vi "GameDataToFieldState.vi"(1 "Game Data":T1={"Close  Switch"=enum."Right", "Scale"=enum."Right", "Far Switch"=enum."Right"}) -> (0 "FieldState":T3)   [LabVIEW 2017]
uses:
  TypeDef/AutoFieldState.ctl
  TypeDef/Game_Data.ctl
  TypeDef/Plate_Positions.ctl
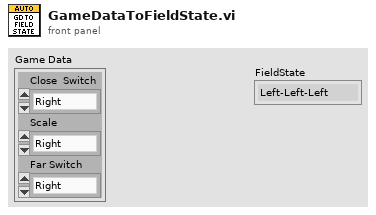
[diagram p1: front panel]
types:
  T1 = typedef "Game_Data.ctl" = cluster{"Close  Switch":T2, "Scale":T2, "Far Switch":T2}
  T2 = typedef "Plate_Positions.ctl" = enum16{"Left", "Right", "Unknown"}
  T3 = typedef "AutoFieldState.ctl" = enum16{"Left-Left-Left", "Left-Right-Left", "Right-Left-Right", "Right-Right-Right", "Unknown"}
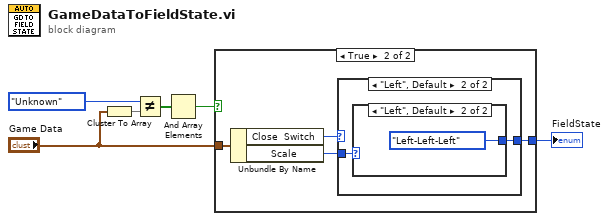
[diagram p0: block diagram]
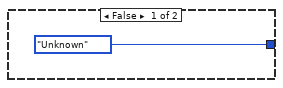
[diagram p2: hidden frame]
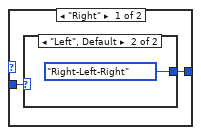
[diagram p3: hidden frame]
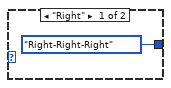
[diagram p4: hidden frame]
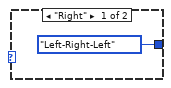
[diagram p5: hidden frame]
diagram:
  n1 = Cluster To Array(cluster="Game Data") -> (array=w5:T2[])
  n2 = Not Equal?(x=Plate_Positions."Unknown" ("Plate Position"), y=w5) -> (x != y?=w4:bool[])
  n3 = And Array Elements(Boolean array=w4) -> (logical AND=w3:bool)
  n4 = case shown="True" w3 {
    tunnel: [AutoFieldState."Unknown" ("FieldState") w8] -> w2
    tunnel: "Game Data" -> [_ w11]
    frame False {
    }
    frame True {
      n5 = Unbundle By Name(w11) -> ("Close  Switch"=w10:T2, "Scale"=w9:T2)
      n6 = case shown="\"Left\", Default" w10 {
        tunnel: w9 -> [w13 w17]
        tunnel: [w12 w16] -> w8
        frame "Right" {
          n7 = case shown="\"Left\", Default" w13 {
            tunnel: [AutoFieldState."Right-Right-Right" ("FieldState") AutoFieldState."Right-Left-Right" ("FieldState")] -> w12
            frame "Right" {
            }
            frame "Left", Default {
            }
          }
        }
        frame "Left", Default {
          n8 = case shown="\"Left\", Default" w17 {
            tunnel: [AutoFieldState."Left-Right-Left" ("FieldState") AutoFieldState."Left-Left-Left" ("FieldState")] -> w16
            frame "Right" {
            }
            frame "Left", Default {
            }
          }
        }
      }
    }
  }
  "FieldState" <- w2
